vi "Popup - Main Menu.vi"(8 "error in":errorcluster) -> (0 "error out":errorcluster, 1 "IsNewTest":bool, 2 "FuelFarm":bool, 3 "Exit":bool)   [LabVIEW 2018, in "Controller (Host).lvlib"]
doc: "This is the dialog used by the user to select an APU to test."
uses:
  Controller (Host).lvlib
panel:
  in  "FuelFarm":bool
  in  "Continue Test":bool
  in  "Exit":bool
  in  "New Test":bool
  # "APU TEST CELL"
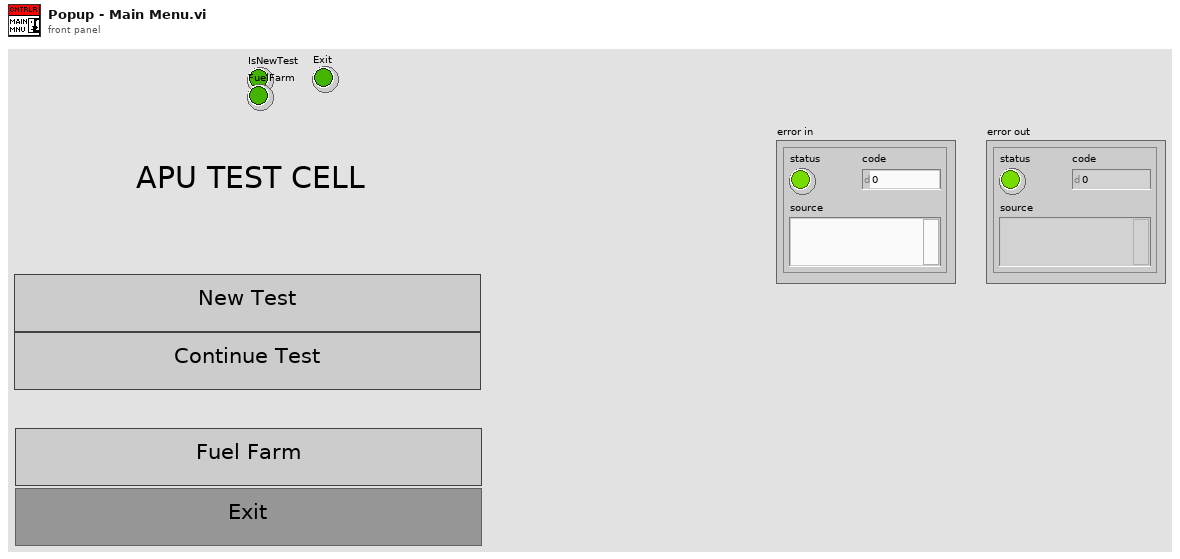
[diagram p1: front panel]
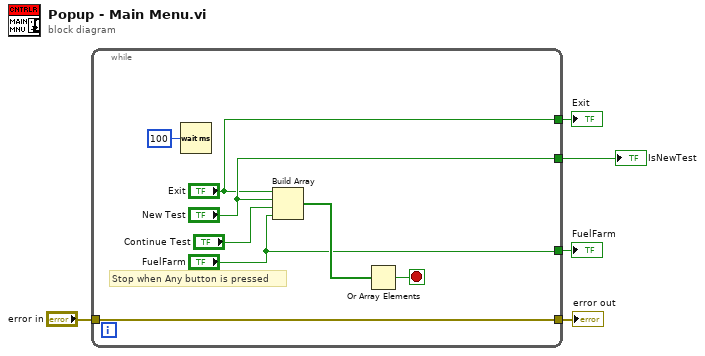
[diagram p0: block diagram]
diagram:
  n1 = while {
    tunnel: "error in" -> [w12]
    tunnel: [w12] -> w4
    tunnel: ["New Test"] -> w3
    tunnel: ["Exit"] -> w2
    tunnel: ["FuelFarm"] -> w1
    stop <- w10 stop-if-true
    # "Stop when Any button is pressed"
    n2 = Wait (ms)(milliseconds to wait=u32 100) -> ()  [unwired: 1 out]
    n3 = Build Array("Exit", "New Test", "Continue Test", "FuelFarm") -> (w11:bool[])
    n4 = Or Array Elements(Boolean array=w11) -> (logical OR=w10:bool)
  }
  "error out" <- w4
  "IsNewTest" <- w3
  "Exit" <- w2
  "FuelFarm" <- w1
